vi "Terminate.vi"(8 "error in (no error)":errorcluster, 10 "Message in":refnum<class "TerminateMessage.lvclass">, 11 "DAQMH121119OrcaFlash in":refnum<class "DAQOrcaFlash.lvclass">) -> (0 "error out":errorcluster, 3 "DAQMH121119OrcaFlash out":refnum<class "DAQOrcaFlash.lvclass">)   [LabVIEW 2012, in "DAQOrcaFlash.lvclass"]
doc: "This member function is called when the statemachine in the run.vi receives an 'terminate' command. It closes the RabbitMQ connection. \n\nOverride this member function in your derived class to release all previously acquired resources (but don't forget to call the parent method). If your component has subcomponents, they count as resources, and you have to release them by calling their own terminate functions."
uses:
  DAQOrcaFlash.lvclass
  <vilib>/Distrio/Murmex/TerminateMessage/TerminateMessage.lvclass
  <vilib>/Distrio/Murmex/StopMessage/StopMessage.lvclass
  DAQOrcaFlash.lvclass/DAQOrcaFlash.ctl
  <vilib>/Distrio/Murmex/Murmex/Murmex.lvclass
panel:
  # "This method is called when the TERMINATE\ntrigger is sent. \n\nOverride this method when your component needs to\nrespond to this trigger. \n\nCall parent for proper implementation"
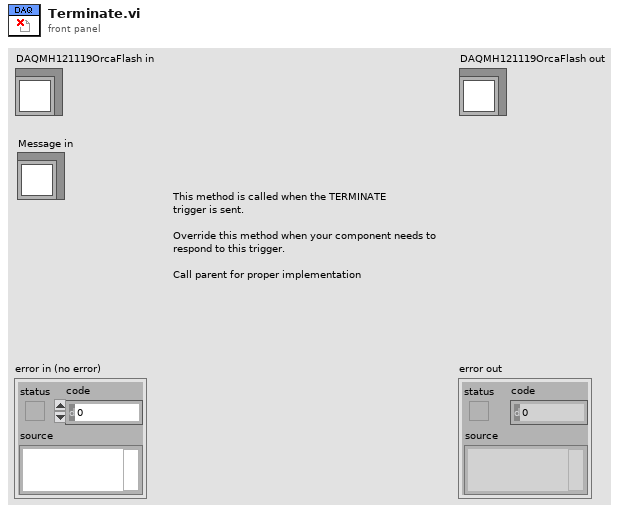
[diagram p1: front panel]
types:
  T1 = typedef "IMAQ Image.ctl" = refnum<image>
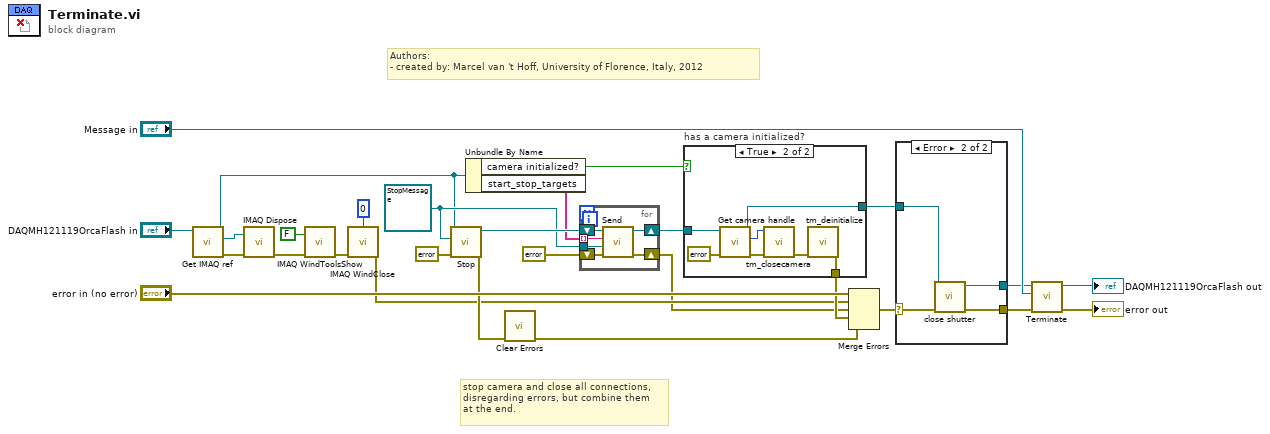
[diagram p0: block diagram]
diagram:
  w10 = refnum<class "StopMessage.lvclass"> refnum ("Message in")
  # "stop camera and close all connections,\ndisregarding errors, but combine them\nat the end."
  # "Authors: \n- created by: Marcel van 't Hoff, University of Florence, Italy, 2012"
  n1 = call "Get IMAQ ref.vi"("DAQMH121119OrcaFlash in"="DAQMH121119OrcaFlash in") -> ("error out"=w20:errorcluster, "IMAQ reference"=w21:T1, "DAQMH121119OrcaFlash out"=w9:refnum<class "DAQOrcaFlash.lvclass">)  [unwired: 8 in]
  n2 = call "IMAQ Dispose"("Image"=w21, "error in (no error)"=w20) -> ("error out"=w19:errorcluster)  [unwired: 4 in]
  n3 = call "IMAQ WindToolsShow"("Hide/Show (Show)"=FALSE, "error in (no error)"=w19) -> ("error out"=w18:errorcluster)  [unwired: 3 in, 1 out]
  n4 = call "IMAQ WindClose"("Window Number (0...15)"=0, "error in (no error)"=w18) -> ("error out"=w16:errorcluster)  [unwired: 4 in]
  n5 = call-dynamic "Stop.vi"("error in (no error)"=errorcluster {"status"=FALSE, "code"=0, "source"=""}, "Message in"=w10, "DAQMH121119OrcaFlash in"=w9) -> ("error out"=w25:errorcluster, "DAQMH121119OrcaFlash out"=w15:refnum<class "DAQOrcaFlash.lvclass">)  [unwired: 7 in]
  n6 = Unbundle By Name(w9) -> ("camera initialized?"=w8:bool, "start_stop_targets"=w12:string[])
  n7 = call <vilib>:"Clear Errors.vi"("error in (no error)"=w25) -> ("error out"=w23:errorcluster)  [unwired: 6 in]
  n8 = for {
    tunnel: w12 -> [w31] mode=indexing
    shift-right: [w33] -> w14
    shift-left: w15 -> [w34]
    shift-right: [w30] -> w11
    shift-left: errorcluster {"status"=FALSE, "code"=0, "source"=""} ("error in (no error)") -> [w32]
    tunnel: w10 -> [w29]
    n9 = call <vilib>:"Send.vi"("error in (no error)"=w32, "Message"=w29, "recipient"=w31, "Murmex in"=w34) -> ("error out"=w30:errorcluster, "Murmex out"=w33:refnum<class "DAQOrcaFlash.lvclass">)  [unwired: 6 in]
  }
  n10 = case "has a camera initialized?" shown="True" w8 {
    tunnel: [w35 w42] -> w6
    tunnel: [_ w37] -> w24
    tunnel: w14 -> [w35 w36]
    frame False {
    }
    frame True {
      n11 = call "Get camera handle.vi"("error in (no error)"=errorcluster {"status"=FALSE, "code"=0, "source"=""}, "DAQMH121119OrcaFlash in"=w36) -> ("error out"=w39:errorcluster, "cam handle"=w40:u32, "DAQMH121119OrcaFlash out"=w42:refnum<class "DAQOrcaFlash.lvclass">)  [unwired: 7 in]
      n12 = call <userlib>:"tm_closecamera.vi"("error in (no error)"=w39, "Handle in"=w40) -> ("error out"=w41:errorcluster)  [unwired: 9 in]
      n13 = call <userlib>:"tm_deinitialize.vi"("error in (no error)"=w41) -> ("error out"=w37:errorcluster)  [unwired: 10 in]
    }
  }
  n14 = Merge Errors("error in (no error)", w16, w11, w24, w23) -> (w7:errorcluster)
  n15 = case shown="Error" w7 {
    selector: w7 -> [w44 w48]
    tunnel: [w44 w47] -> w4
    tunnel: w6 -> [w43 w46]
    tunnel: [w43 w45] -> w1
    frame No Error {
    }
    frame Error {
      n16 = call "close shutter.vi"("error in (no error)"=w48, "Murmex in"=w46) -> ("error out"=w47:errorcluster, "Murmex out"=w45:refnum<class "DAQOrcaFlash.lvclass">)  [unwired: 8 in]
    }
  }
  n17 = call-parent "Terminate.vi"("error in (no error)"=w4, "Message in"="Message in", "Murmex in"=w1) -> ("error out"=→"error out":errorcluster, "Murmex out"=→"DAQMH121119OrcaFlash out":refnum<class "DAQOrcaFlash.lvclass">)  [unwired: 7 in]
